vi "Timer.vi"(5 "StateTimer":T1, 11 "Setpoint":i32) -> (0 "Running":bool, 1 "Done":bool, 3 "Time":dbl)   [LabVIEW 2014, in "Master.lvclass"]
uses:
  Master/Master.lvclass
  Controls/StateTimer.ctl
  Controls/Control Library.lvlib
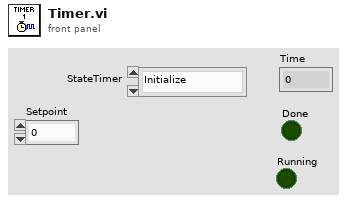
[diagram p1: front panel]
types:
  T1 = typedef "Control Library.lvlib/StateTimer.ctl" = enum16{"Initialize", "RealTime", "Pause", "Stop"}
  T2 = typedef "LVDateTimeRec.ctl" = cluster{"fractional second":dbl, "second":i32, "minute":i32, "hour":i32, "day of month":i32, "month":i32, "year":i32, "day of week":i32, "day of year":i32, "DST":i32}
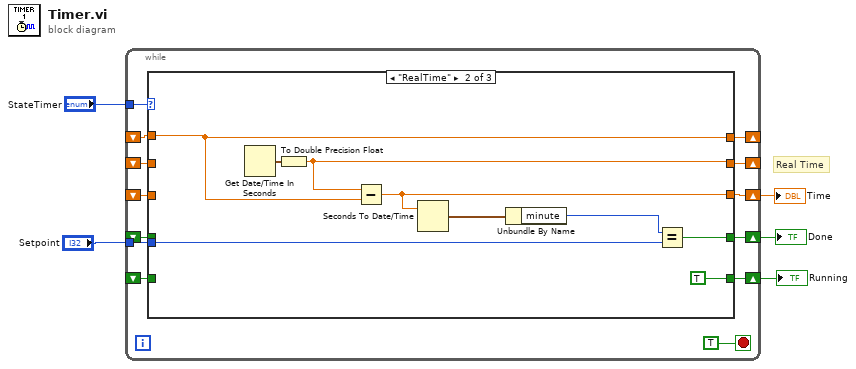
[diagram p0: block diagram]
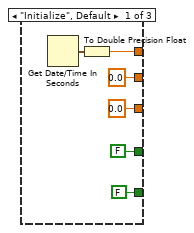
[diagram p2: hidden frame]
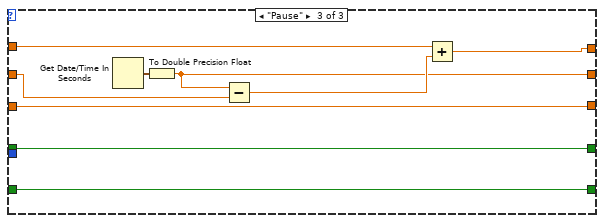
[diagram p3: hidden frame]
diagram:
  # "Real Time"
  n1 = while {
    tunnel: "StateTimer" -> [w17]
    shift-right: [w16] -> _
    shift-left: _ -> [w15]
    shift-right: [w13] -> _
    shift-left: _ -> [w11]
    shift-right: [w12] -> w3
    shift-left: _ -> [w10]
    shift-right: [w14] -> w4
    shift-left: _ -> [w9]
    shift-right: [w8] -> w2
    shift-left: _ -> [w7]
    tunnel: "Setpoint" -> [w6]
    stop <- TRUE stop-if-true
    n2 = case shown="\"RealTime\"" w17 {
      tunnel: [w23 w32 w38] -> w16
      tunnel: w15 -> [_ w32 w40]
      tunnel: [FALSE w31 w35] -> w14
      tunnel: [0.0 w30 w37] -> w13
      tunnel: [0.0 w28 w36] -> w12
      tunnel: w11 -> [_ _ w41]
      tunnel: w10 -> [_ _ w36]
      tunnel: w9 -> [_ _ w35]
      tunnel: [FALSE TRUE w34] -> w8
      tunnel: w7 -> [_ _ w34]
      tunnel: w6 -> [_ w25 _]
      frame "Initialize", Default {
        n3 = Get Date/Time In Seconds() -> (seconds since 1Jan1904=w24:timestamp)
        n4 = To Double Precision Float(number=w24) -> (double precision float=w23:dbl)
      }
      frame "RealTime" {
        n5 = Get Date/Time In Seconds() -> (seconds since 1Jan1904=w33:timestamp)
        n6 = To Double Precision Float(number=w33) -> (double precision float=w30:dbl)
        n7 = Subtract(x=w30, y=w32) -> (x-y=w28:dbl)
        n8 = Seconds To Date/Time(time stamp (now)=w28) -> (date time rec=w27:T2)  [unwired: 1 in]
        n9 = Unbundle By Name(w27) -> ("minute"=w26:i32)
        n10 = Equal?(x=w26, y=w25) -> (x = y?=w31:bool)
      }
      frame "Pause" {
        n11 = Get Date/Time In Seconds() -> (seconds since 1Jan1904=w42:timestamp)
        n12 = To Double Precision Float(number=w42) -> (double precision float=w37:dbl)
        n13 = Subtract(x=w37, y=w41) -> (x-y=w39:dbl)
        n14 = Add(x=w40, y=w39) -> (x+y=w38:dbl)
      }
    }
  }
  "Done" <- w4
  "Time" <- w3
  "Running" <- w2
